vi "Global_SM Write_Data Out.vi"() -> ()   [LabVIEW 2016, in "WC_Drive.lvlib"]
uses:
  WC_Drive.lvlib
  TypeDef/ENUM_Drive_ACT Loop_Mode.ctl
  TypeDef/ENUM_Drive_Profile_CMD.ctl
  TypeDef/CLUSTER_Left and Right.ctl
panel:
  in  "WC_Drive_SM_VBus":T1
  in  "WC_Drive_SM_ProfileCmd":T2
  in  "WC_Drive_SM_Mode":T3
  # "The Names of the Data items in the Global Variable MUST describe who the Single Writer is\nNaming Convention of all Data Items is:   Lib Name_Loop Name (SM or SEN or ACT)_Data Name\nExample   Drive_ACT_X axis;  GameController_SEN_JoystickLeft;  Hopper_SM_AgitatorSpeed"
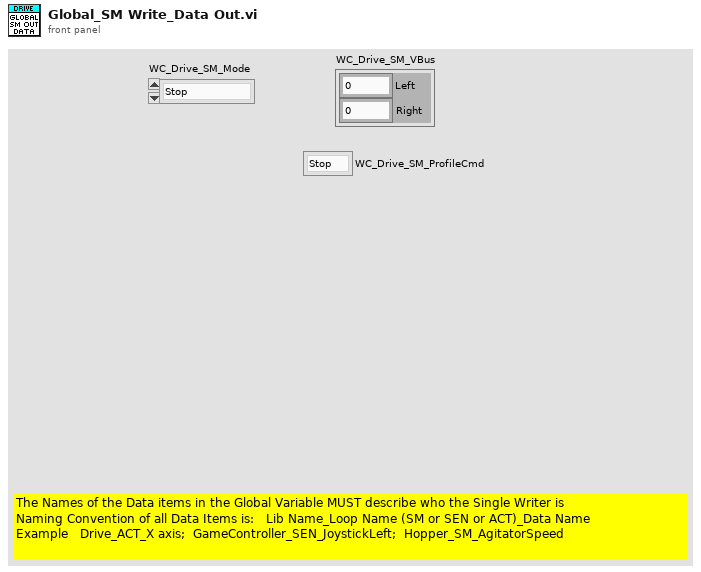
[diagram p1: front panel]
types:
  T1 = typedef "CLUSTER_Left and Right.ctl" = cluster{"Left":dbl, "Right":dbl}
  T2 = typedef "ENUM_Drive_Profile_CMD.ctl" = enum16{"Stop", "Setup", "Run"}
  T3 = typedef "ENUM_Drive_ACT Loop_Mode.ctl" = enum16{"Stop", "VBus", "Profile"}
diagram:
